vi "ASI_serialLEDControl.vi"(2 "Delay Time (s)":dbl, 3 "error in (no error)":errorcluster, 4 "VISA resource name":refnum<visa-resource-name>="COM7", 5 "setpoint":dbl) -> (0 "error out":errorcluster, 1 "VISA resource name out":refnum<visa-resource-name>)   [LabVIEW 2015]
doc: "Establishes connection with configured port (default = COM1).\nSends command MOVE X=x Y=y where x and y are integers denoting 10ths of a micron.\nSub-VI SerialWaitForStatusN.vi polls controller with STATUS command until 'N' (not busy) status is returned, or until a configured maximum number of unsuccessful tries (default = 400).\nDisconnects from configured port."
uses:
  <vilib>/Instr/_visa.llb/VISA Flush IO Buffer Mask.ctl
  GLOBAL/Global_ASI_stage.vi
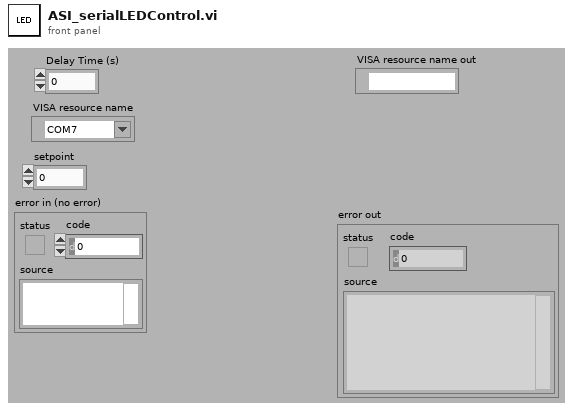
[diagram p1: front panel]
types:
  T1 = typedef "VISA Flush IO Buffer Mask.ctl" = u16
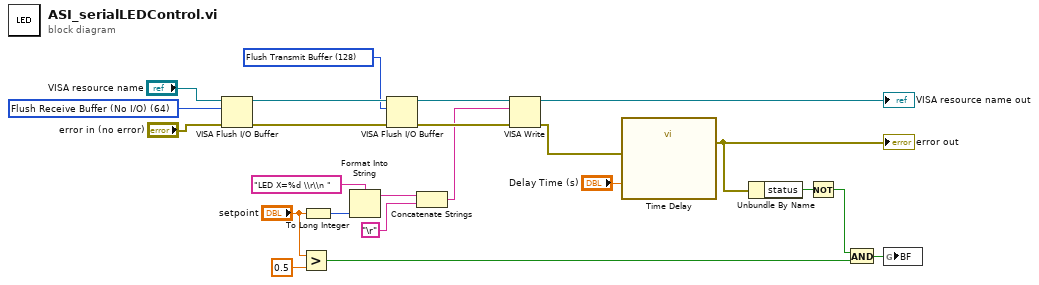
[diagram p0: block diagram]
diagram:
  w18 = T1 128 items=["Flush Receive Buffer"=16, "Write Transmit Buffer to Device"=32, "Flush Receive Buffer (No I/O)"=64, "Flush Transmit Buffer"=128] ("Mask")
  w21 = T1 64 items=["Flush Receive Buffer"=16, "Write Transmit Buffer to Device"=32, "Flush Receive Buffer (No I/O)"=64, "Flush Transmit Buffer"=128] ("Mask")
  n1 = VISA Flush I/O Buffer(VISA resource name="VISA resource name", mask (16)=w21, error in (no error)="error in (no error)") -> (VISA resource name out=w19:refnum<visa-resource-name>, error out=w20:errorcluster)
  n2 = Greater?(x="setpoint", y=0.5) -> (0:w3:bool)
  n3 = To Long Integer(number="setpoint") -> (32bit integer=w7:i32)
  n4 = Format Into String(format string="LED X=%d \\r\\n ", w7) -> (resulting string=w12:string)  [unwired: 2 in, 1 out]
  n5 = VISA Flush I/O Buffer(VISA resource name=w19, mask (16)=w18, error in (no error)=w20) -> (VISA resource name out=w16:refnum<visa-resource-name>, error out=w17:errorcluster)
  n6 = Concatenate Strings(w12, "\r") -> (w11:string)
  n7 = VISA Write(VISA resource name=w16, write buffer=w11, error in (no error)=w17) -> (VISA resource name out=→"VISA resource name out":refnum<visa-resource-name>, error out=w14:errorcluster)  [unwired: 1 out]
  n8 = call "Time Delay"("error in (no error)"=w14, "Delay Time (s)"="Delay Time (s)") -> ("error out"=w1:errorcluster)  [unwired: 9 in]
  "error out" <- w1
  n9 = Unbundle By Name(w1) -> ("status"=w4:bool)
  n10 = Not(x=w4) -> (.not. x?=w5:bool)
  n11 = And(x=w5, y=w3) -> (x .and. y?=w6:bool)
  n12 = global write "Global_ASI_stage.vi" "BF"(w6) -> ()
